vi "test_read-nmea-data2.vi"() -> ()   [LabVIEW 2019] (continued)
104,,19,25,045,,25,08,248,,36,27,309,,2*77\n\t\n15:15:25.65\tF9P\t$GBGSV,2,1,06,07,,,26,11,48,133,32,14,87,101,33,28,,,24,1*7A\n\t\n15:15:25.67\tF9P\t$GBGSV,2,2,06,33,62,220,35,34,,,26,1*41\n\t\n15:15:25.69\tF9P\t$GBGSV,1,1,03,11,48,133,33,14,87,101,29,33,62,220,,3*4F\n\t\n15:15:25.71\tF9P\t$GNGLL,3723.59755,N,12656.93215,E,061527.00,A,A*74\n\t\n15:15:25.73\tF9P\t\t\n15:15:25.75\tF9P\t\t\n15:15:25.77\tF9P\t\t\n15:15:25.79\tF9P\t\t\n15:15:25.81\tF9P\t\t\n15:15:25.83\tF9P\t\t\n15:15:25.85\tF9P\t\t\n15:15:25.87\tF9P\t\t\n15:15:25.89\tF9P\t\t\n15:15:25.91\tF9P\t\t\n15:15:25.93\tF9P\t\t\n15:15:25.95\tF9P\t\t\n15:15:25.97\tF9P\t\t\n15:15:25.99\tF9P\t\t\n15:15:26.01\tF9P\t\t\n15:15:26.03\tF9P\t\t\n15:15:26.05\tF9P\t\t\n15:15:26.07\tF9P\t\t\n15:15:26.09\tF9P\t\t\n15:15:26.11\tF9P\t\t\n15:15:26.13\tF9P\t\t\n15:15:26.15\tF9P\t\t\n15:15:26.17\tF9P\t\t\n15:15:26.19\tF9P\t\t\n15:15:26.21\tF9P\t\t\n15:15:26.23\tF9P\t$GNRMC,061528.00,A,3723.59768,N,12656.93177,E,0.064,,250720,,,A,V*11\n\t\n15:15:26.25\tF9P\t$GNVTG,,T,,M,0.064,N,0.118,K,A*37\n\t\n15:15:26.27\tF9P\t$GNGGA,061528.00,3723.59768,N,12656.93177,E,1,12,0.80,45.8,M,18.5,M,,*79\n\t\n15:15:26.29\tF9P\t$GNGSA,A,3,12,06,19,05,17,09,04,02,,,,,1.41,0.80,1.16,1*0A\n\t\n15:15:26.31\tF9P\t$GNGSA,A,3,85,70,71,84,,,,,,,,,1.41,0.80,1.16,2*08\n\t\n15:15:26.33\tF9P\t$GNGSA,A,3,36,19,11,04,09,12,,,,,,,1.41,0.80,1.16,3*0A\n\t\n15:15:26.35\tF9P\t$GNGSA,A,3,14,11,33,,,,,,,,,,1.41,0.80,1.16,4*0B\n\t\n15:15:26.37\tF9P\t$GPGSV,3,1,09,02,56,320,21,04,17,043,28,05,38,248,29,06,64,051,33,1*68\n\t\n15:15:26.39\tF9P\t$GPGSV,3,2,09,09,44,072,32,12,23,275,40,17,31,154,26,19,51,157,27,1*6D\n\t\n15:15:26.41\tF9P\t$GPGSV,3,3,09,25,12,305,21,1*5C\n\t\n15:15:26.43\tF9P\t$GPGSV,3,1,09,02,56,320,,04,17,043,18,05,38,248,22,06,64,051,30,6*67\n\t\n15:15:26.45\tF9P\t$GPGSV,3,2,09,09,44,072,26,12,23,275,21,17,31,154,,19,51,157,,6*69\n\t\n15:15:26.47\tF9P\t$GPGSV,3,3,09,25,12,305,,6*58\n\t\n15:15:26.49\tF9P\t$GLGSV,2,1,08,69,10,031,21,70,70,037,34,71,54,207,37,72,05,210,,1*7A\n\t\n15:15:26.51\tF9P\t$GLGSV,2,2,08,77,01,324,,84,19,123,10,85,69,072,37,86,38,331,,1*76\n\t\n15:15:26.53\tF9P\t$GLGSV,2,1,08,69,10,031,13,70,70,037,,71,54,207,31,72,05,210,,3*78\n\t\n15:15:26.55\tF9P\t$GLGSV,2,2,08,77,01,324,,84,19,123,11,85,69,072,34,86,38,331,,3*76\n\t\n15:15:26.57\tF9P\t$GAGSV,2,1,08,02,08,296,11,04,67,114,40,09,33,193,28,11,72,002,35,7*73\n\t\n15:15:26.59\tF9P\t$GAGSV,2,2,08,12,39,104,26,19,25,044,26,25,08,248,,36,27,309,18,7*7A\n\t\n15:15:26.61\tF9P\t$GAGSV,2,1,08,02,08,296,,04,67,114,,09,33,193,,11,72,002,33,2*7E\n\t\n15:15:26.63\tF9P\t$GAGSV,2,2,08,12,39,104,,19,25,044,,25,08,248,,36,27,309,,2*76\n\t\n15:15:26.65\tF9P\t$GBGSV,2,1,06,07,,,25,11,48,133,32,14,87,101,35,28,,,24,1*7F\n\t\n15:15:26.67\tF9P\t$GBGSV,2,2,06,33,62,220,36,34,,,26,1*42\n\t\n15:15:26.69\tF9P\t$GBGSV,1,1,03,11,48,133,,14,87,101,23,33,62,220,,3*45\n\t\n15:15:26.71\tF9P\t$GNGLL,3723.59768,N,12656.93177,E,061528.00,A,A*72\n\t\n15:15:26.73\tF9P\t\t\n15:15:26.75\tF9P\t\t\n15:15:26.77\tF9P\t\t\n15:15:26.79\tF9P\t\t\n15:15:26.81\tF9P\t\t\n15:15:26.83\tF9P\t\t\n15:15:26.85\tF9P\t\t\n15:15:26.87\tF9P\t\t\n15:15:26.89\tF9P\t\t\n15:15:26.91\tF9P\t\t\n15:15:26.93\tF9P\t\t\n15:15:26.95\tF9P\t\t\n15:15:26.97\tF9P\t\t\n15:15:26.99\tF9P\t\t\n15:15:27.01\tF9P\t\t\n15:15:27.03\tF9P\t\t\n15:15:27.05\tF9P\t\t\n15:15:27.07\tF9P\t\t\n15:15:27.09\tF9P\t\t\n15:15:27.11\tF9P\t\t\n15:15:27.13\tF9P\t\t\n15:15:27.15\tF9P\t\t\n15:15:27.17\tF9P\t\t\n15:15:27.19\tF9P\t\t\n15:15:27.21\tF9P\t\t\n15:15:27.23\tF9P\t$GNRMC,061529.00,A,3723.59788,N,12656.93143,E,0.112,,250720,,,A,V*19\n\t\n15:15:27.25\tF9P\t$GNVTG,,T,,M,0.112,N,0.208,K,A*35\n\t\n15:15:27.27\tF9P\t$GNGGA,061529.00,3723.59788,N,12656.93143,E,1,12,0.72,45.7,M,18.5,M,,*73\n\t\n15:15:27.29\tF9P\t$GNGSA,A,3,12,06,19,05,17,09,04,02,,,,,1.23,0.72,1.00,1*04\n\t\n15:15:27.31\tF9P\t$GNGSA,A,3,85,70,71,84,,,,,,,,,1.23,0.72,1.00,2*06\n\t\n15:15:27.33\tF9P\t$GNGSA,A,3,36,19,11,04,09,12,,,,,,,1.23,0.72,1.00,3*04\n\t\n15:15:27.35\tF9P\t$GNGSA,A,3,14,11,33,,,,,,,,,,1.23,0.72,1.00,4*05\n\t\n15:15:27.37\tF9P\t$GPGSV,3,1,09,02,56,320,21,04,17,043,28,05,38,248,29,06,64,051,33,1*68\n\t\n15:15:27.39\tF9P\t$GPGSV,3,2,09,09,44,072,36,12,23,275,39,17,31,154,25,19,51,157,27,1*64\n\t\n15:15:27.41\tF9P\t$GPGSV,3,3,09,25,12,305,23,1*5E\n\t\n15:15:27.43\tF9P\t$GPGSV,3,1,09,02,56,320,,04,17,043,18,05,38,248,22,06,64,051,30,6*67\n\t\n15:15:27.45\tF9P\t$GPGSV,3,2,09,09,44,072,27,12,23,275,15,17,31,154,,19,51,157,,6*6F\n\t\n15:15:27.47\tF9P\t$GPGSV,3,3,09,25,12,305,,6*58\n\t\n15:15:27.49\tF9P\t$GLGSV,2,1,08,69,10,031,22,70,70,037,29,71,54,207,30,72,05,210,,1*72\n\t\n15:15:27.51\tF9P\t$GLGSV,2,2,08,77,01,324,,84,19,123,12,85,69,072,38,86,38,331,,1*7B\n\t\n15:15:27.53\tF9P\t$GLGSV,2,1,08,69,10,031,13,70,70,037,,71,54,207,30,72,05,210,,3*79\n\t\n15:15:27.55\tF9P\t$GLGSV,2,2,08,77,01,324,,84,19,123,10,85,69,072,28,86,38,331,,3*7A\n\t\n15:15:27.57\tF9P\t$GAGSV,2,1,08,02,08,296,07,04,67,114,42,09,33,193,28,11,72,002,34,7*77\n\t\n15:15:27.59\tF9P\t$GAGSV,2,2,08,12,39,104,26,19,25,044,25,25,08,248,,36,27,309,11,7*70\n\t\n15:15:27.61\tF9P\t$GAGSV,2,1,08,02,08,296,,04,67,114,30,09,33,193,,11,72,002,32,2*7C\n\t\n15:15:27.63\tF9P\t$GAGSV,2,2,08,12,39,104,,19,25,044,,25,08,248,,36,27,309,,2*76\n\t\n15:15:27.65\tF9P\t$GBGSV,2,1,06,07,,,25,11,48,133,33,14,87,101,31,28,,,20,1*7E\n\t\n15:15:27.67\tF9P\t$GBGSV,2,2,06,33,62,220,38,34,,,27,1*4D\n\t\n15:15:27.69\tF9P\t$GBGSV,1,1,03,11,48,133,,14,87,101,,33,62,220,,3*44\n\t\n15:15:27.71\tF9P\t$GNGLL,3723.59788,N,12656.93143,E,061529.00,A,A*7A\n\t\n15:15:27.73\tF9P\t\t\n15:15:27.75\tF9P\t\t\n15:15:27.77\tF9P\t\t\n15:15:27.79\tF9P\t\t\n15:15:27.81\tF9P\t\t\n15:15:27.83\tF9P\t\t\n15:15:27.85\tF9P\t\t\n15:15:27.87\tF9P\t\t\n15:15:27.89\tF9P\t\t\n15:15:27.91\tF9P\t\t\n15:15:27.93\tF9P\t\t\n15:15:27.95\tF9P\t\t\n15:15:27.97\tF9P\t\t\n15:15:27.99\tF9P\t\t\n15:15:28.01\tF9P\t\t\n15:15:28.03\tF9P\t\t\n15:15:28.05\tF9P\t\t\n15:15:28.07\tF9P\t\t\n15:15:28.09\tF9P\t\t\n15:15:28.11\tF9P\t\t\n15:15:28.13\tF9P\t\t\n15:15:28.15\tF9P\t\t\n15:15:28.17\tF9P\t\t\n15:15:28.19\tF9P\t\t\n15:15:28.21\tF9P\t\t\n15:15:28.23\tF9P\t$GNRMC,061530.00,A,3723.59812,N,12656.93103,E,0.030,,250720,,,A,V*18\n\t\n15:15:28.25\tF9P\t$GNVTG,,T,,M,0.030,N,0.055,K,A*3E\n\t\n15:15:28.27\tF9P\t$GNGGA,061530.00,3723.59812,N,12656.93103,E,1,12,0.71,45.7,M,18.5,M,,*70\n\t\n15:15:28.29\tF9P\t$GNGSA,A,3,12,06,19,05,17,09,04,02,,,,,1.22,0.71,1.00,1*06\n\t\n15:15:28.31\tF9P\t$GNGSA,A,3,85,70,71,84,,,,,,,,,1.22,0.71,1.00,2*04\n\t\n15:15:28.33\tF9P\t$GNGSA,A,3,36,19,11,04,09,12,,,,,,,1.22,0.71,1.00,3*06\n\t\n15:15:28.35\tF9P\t$GNGSA,A,3,14,11,33,,,,,,,,,,1.22,0.71,1.00,4*07\n\t\n15:15:28.37\tF9P\t$GPGSV,3,1,09,02,56,320,20,04,17,043,26,05,38,248,28,06,64,051,33,1*66\n\t\n15:15:28.39\tF9P\t$GPGSV,3,2,09,09,44,072,35,12,23,275,37,17,31,154,24,19,51,157,27,1*68\n\t\n15:15:28.41\tF9P\t$GPGSV,3,3,09,25,12,305,25,1*58\n\t\n15:15:28.43\tF9P\t$GPGSV,3,1,09,02,56,320,,04,17,043,18,05,38,248,22,06,64,051,32,6*65\n\t\n15:15:28.45\tF9P\t$GPGSV,3,2,09,09,44,072,27,12,23,275,16,17,31,154,,19,51,157,,6*6C\n\t\n15:15:28.47\tF9P\t$GPGSV,3,3,09,25,12,305,,6*58\n\t\n15:15:28.49\tF9P\t$GLGSV,2,1,08,69,10,031,22,70,70,037,28,71,54,207,37,72,05,210,,1*74\n\t\n15:15:28.51\tF9P\t$GLGSV,2,2,08,77,01,324,,84,19,123,11,85,69,072,39,86,38,331,,1*79\n\t\n15:15:28.53\tF9P\t$GLGSV,2,1,08,69,10,031,13,70,70,037,,71,54,207,30,72,05,210,,3*79\n\t\n15:15:28.55\tF9P\t$GLGSV,2,2,08,77,01,324,,84,19,123,09,85,69,072,30,86,38,331,,3*7B\n\t\n15:15:28.57\tF9P\t$GAGSV,2,1,08,02,08,296,08,04,67,114,39,09,33,193,33,11,72,002,32,7*78\n\t\n15:15:28.59\tF9P\t$GAGSV,2,2,08,12,39,104,27,19,25,044,22,25,08,248,,36,27,309,13,7*74\n\t\n15:15:28.61\tF9P\t$GAGSV,2,1,08,02,08,296,,04,67,114,34,09,33,193,,11,72,002,32,2*78\n\t\n15:15:28.63\tF9P\t$GAGSV,2,2,08,12,39,104,,19,25,044,,25,08,248,,36,27,309,,2*76\n\t\n15:15:28.65\tF9P\t$GBGSV,2,1,06,07,,,25,11,48,133,32,14,87,101,27,28,,,23,1*7B\n\t\n15:15:28.67\tF9P\t$GBGSV,2,2,06,33,62,220,37,34,,,28,1*4D\n\t\n15:15:28.69\tF9P\t$GBGSV,1,1,03,11,48,133,,14,87,101,,33,62,220,,3*44\n\t\n15:15:28.71\tF9P\t$GNGLL,3723.59812,N,12656.93103,E,061530.00,A,A*7A\n\t\n15:15:28.73\tF9P\t\t\n15:15:28.75\tF9P\t\t\n15:15:28.77\tF9P\t\t\n15:15:28.79\tF9P\t\t\n15:15:28.81\tF9P\t\t\n15:15:28.83\tF9P\t\t\n15:15:28.85\tF9P\t\t\n15:15:28.87\tF9P\t\t\n15:15:28.89\tF9P\t\t\n15:15:28.91\tF9P\t\t\n15:15:28.93\tF9P\t\t\n15:15:28.95\tF9P\t\t\n15:15:28.97\tF9P\t\t\n15:15:28.99\tF9P\t\t\n15:15:29.01\tF9P\t\t\n15:15:29.03\tF9P\t\t\n15:15:29.05\tF9P\t\t\n15:15:29.07\tF9P\t\t\n15:15:29.09\tF9P\t\t\n15:15:29.11\tF9P\t\t\n15:15:29.13\tF9P\t\t\n15:15:29.15\tF9P\t\t\n15:15:29.17\tF9P\t\t\n15:15:29.19\tF9P\t\t\n15:15:29.21\tF9P\t\t\n15:15:29.23\tF9P\t$GNRMC,061531.00,A,3723.59835,N,12656.93068,E,0.052,,250720,,,A,V*14\n\t\n15:15:29.25\tF9P\t$GNVTG,,T,,M,0.052,N,0.096,K,A*35\n\t\n15:15:29.27\tF9P\t$GNGGA,061531.00,3723.59835,N,12656.93068,E,1,12,0.71,45.6,M,18.5,M,,*79\n\t\n15:15:29.29\tF9P\t$GNGSA,A,3,12,06,19,05,17,09,04,02,,,,,1.22,0.71,1.00,1*06\n\t\n15:15:29.31\tF9P\t$GNGSA,A,3,85,70,71,84,,,,,,,,,1.22,0.71,1.00,2*04\n\t\n15:15:29.33\tF9P\t$GNGSA,A,3,36,19,11,04,09,12,,,,,,,1.22,0.71,1.00,3*06\n\t\n15:15:29.35\tF9P\t$GNGSA,A,3,14,11,33,,,,,,,,,,1.22,0.71,1.00,4*07\n\t\n15:15:29.37\tF9P\t$GPGSV,3,1,09,02,56,320,19,04,17,043,27,05,38,248,20,06,64,051,37,1*61\n\t\n15:15:29.39\tF9P\t$GPGSV,3,2,09,09,44,072,26,12,23,275,37,17,31,154,22,19,51,157,27,1*6C\n\t\n15:15:29.41\tF9P\t$GPGSV,3,3,09,25,12,305,25,1*58\n\t\n15:15:29.43\tF9P\t$GPGSV,3,1,09,02,56,320,,04,17,043,19,05,38,248,23,06,64,051,34,6*63\n\t\n15:15:29.45\tF9P\t$GPGSV,3,2,09,09,44,072,27,12,23,275,21,17,31,154,,19,51,157,,6*68\n\t\n15:15:29.47\tF9P\t$GPGSV,3,3,09,25,12,305,,6*58\n\t\n15:15:29.49\tF9P\t$GLGSV,2,1,08,69,10,031,25,70,70,037,32,71,54,207,37,72,05,210,,1*78\n\t\n15:15:29.51\tF9P\t$GLGSV,2,2,08,77,01,324,,84,19,123,11,85,69,072,40,86,38,331,,1*77\n\t\n15:15:29.53\tF9P\t$GLGSV,2,1,08,69,10,031,10,70,70,037,,71,54,207,29,72,05,210,,3*72\n\t\n15:15:29.55\tF9P\t$GLGSV,2,2,08,77,01,324,,84,19,123,12,85,69,072,32,86,38,331,,3*73\n\t\n15:15:29.57\tF9P\t$GAGSV,2,1,08,02,08,296,08,04,67,114,39,09,33,193,30,11,72,002,32,7*7B\n\t\n15:15:29.59\tF9P\t$GAGSV,2,2,08,12,39,104,27,19,25,044,22,25,08,248,,36,27,309,14,7*73\n\t\n15:15:29.61\tF9P\t$GAGSV,2,1,08,02,08,296,,04,67,114,29,09,33,193,,11,72,002,32,2*74\n\t\n15:15:29.63\tF9P\t$GAGSV,2,2,08,12,39,104,,19,25,044,,25,08,248,,36,27,309,,2*76\n\t\n15:15:29.65\tF9P\t$GBGSV,2,1,06,07,,,25,11,48,133,31,14,87,101,30,28,,,23,1*7E\n\t\n15:15:29.67\tF9P\t$GBGSV,2,2,06,33,62,220,37,34,,,28,1*4D\n\t\n15:15:29.69\tF9P\t$GBGSV,1,1,03,11,48,133,,14,87,101,,33,62,220,,3*44\n\t\n15:15:29.71\tF9P\t$GNGLL,3723.59835,N,12656.93068,E,061531.00,A,A*72\n\t\n15:15:29.73\tF9P\t\t\n15:15:29.75\tF9P\t\t\n15:15:29.77\tF9P\t\t\n15:15:29.79\tF9P\t\t\n15:15:29.81\tF9P\t\t\n15:15:29.83\tF9P\t\t\n15:15:29.85\tF9P\t\t\n15:15:29.87\tF9P\t\t\n15:15:29.89\tF9P\t\t\n15:15:29.91\tF9P\t\t\n15:15:29.93\tF9P\t\t\n15:15:29.95\tF9P\t\t\n15:15:29.97\tF9P\t\t\n15:15:29.99\tF9P\t\t\n15:15:30.01\tF9P\t\t\n15:15:30.03\tF9P\t\t\n15:15:30.05\tF9P\t\t\n15:15:30.07\tF9P\t\t\n15:15:30.09\tF9P\t\t\n15:15:30.11\tF9P\t\t\n15:15:30.13\tF9P\t\t\n15:15:30.15\tF9P\t\t\n15:15:30.17\tF9P\t\t\n15:15:30.19\tF9P\t\t\n15:15:30.21\tF9P\t\t\n15:15:30.23\tF9P\t$GNRMC,061532.00,A,3723.59857,N,12656.93043,E,0.021,,250720,,,A,V*1E\n\t\n15:15:30.25\tF9P\t$GNVTG,,T,,M,0.021,N,0.040,K,A*3A\n\t\n15:15:30.27\tF9P\t$GNGGA,061532.00,3723.59857,N,12656.93043,E,1,12,0.71,45.7,M,18.5,M,,*76\n\t\n15:15:30.29\tF9P\t$GNGSA,A,3,12,06,19,05,17,09,04,02,,,,,1.22,0.71,1.00,1*06\n\t\n15:15:30.31\tF9P\t$GNGSA,A,3,85,70,71,84,,,,,,,,,1.22,0.71,1.00,2*04\n\t\n15:15:30.33\tF9P\t$GNGSA,A,3,36,19,11,04,09,12,,,,,,,1.22,0.71,1.00,3*06\n\t\n15:15:30.35\tF9P\t$GNGSA,A,3,14,11,33,,,,,,,,,,1.22,0.71,1.00,4*07\n\t\n15:15:30.37\tF9P\t$GPGSV,3,1,09,02,56,320,21,04,17,043,28,05,38,248,30,06,64,051,36,1*65\n\t\n15:15:30.39\tF9P\t$GPGSV,3,2,09,09,44,072,25,12,23,275,36,17,31,154,19,19,51,157,29,1*68\n\t\n15:15:30.41\tF9P\t$GPGSV,3,3,09,25,12,305,26,1*5B\n\t\n15:15:30.43\tF9P\t$GPGSV,3,1,09,02,56,320,,04,17,043,18,05,38,248,23,06,64,051,33,6*65\n\t\n15:15:30.45\tF9P\t$GPGSV,3,2,09,09,44,072,27,12,23,275,24,17,31,154,,19,51,157,,6*6D\n\t\n15:15:30.47\tF9P\t$GPGSV,3,3,09,25,12,305,,6*58\n\t\n15:15:30.49\tF9P\t$GLGSV,2,1,08,69,10,031,28,70,70,037,33,71,54,207,33,72,05,210,,1*70\n\t\n15:15:30.51\tF9P\t$GLGSV,2,2,08,77,01,324,,84,19,123,11,85,69,072,40,86,38,331,,1*77\n\t\n15:15:30.53\tF9P\t$GLGSV,2,1,08,69,10,031,08,70,70,037,,71,54,207,29,72,05,210,,3*7B\n\t\n15:15:30.55\tF9P\t$GLGSV,2,2,08,77,01,324,,84,19,123,16,85,69,072,33,86,38,331,,3*76\n\t\n15:15:30.57\tF9P\t$GAGSV,2,1,08,02,08,296,11,04,67,114,39,09,33,193,32,11,72,002,31,7*72\n\t\n15:15:30.59\tF9P\t$GAGSV,2,2,08,12,39,104,27,19,25,044,21,25,08,248,,36,27,309,13,7*77\n\t\n15:15:30.61\tF9P\t$GAGSV,2,1,08,02,08,296,,04,67,114,27,09,33,193,27,11,72,002,33,2*7E\n\t\n15:15:30.63\tF9P\t$GAGSV,2,2,08,12,39,104,,19,25,044,,25,08,248,,36,27,309,,2*76\n\t\n15:15:30.65\tF9P\t$GBGSV,2,1,06,07,,,23,11,48,133,30,14,87,101,31,28,,,25,1*7E\n\t\n15:15:30.67\tF9P\t$GBGSV,2,2,06,33,62,220,38,34,,,28,1*42\n\t\n15:15:30.69\tF9P\t$GBGSV,1,1,03,11,48,133,,14,87,101,,33,62,220,,3*44\n\t\n15:15:30.71\tF9P\t$GNGLL,3723.59857,N,12656.93043,E,061532.00,A,A*7C\n\t\n15:15:30.73\tF9P\t\t\n15:15:30.75\tF9P\t\t\n15:15:30.77\tF9P\t\t\n15:15:30.79\tF9P\t\t\n15:15:30.81\tF9P\t\t\n15:15:30.83\tF9P\t\t\n15:15:30.85\tF9P\t\t\n15:15:30.87\tF9P\t\t\n15:15:30.89\tF9P\t\t\n15:15:30.91\tF9P\t\t\n15:15:30.93\tF9P\t\t\n15:15:30.95\tF9P\t\t\n15:15:30.97\tF9P\t\t\n15:15:30.99\tF9P\t\t\n15:15:31.01\tF9P\t\t\n15:15:31.03\tF9P\t\t\n15:15:31.05\tF9P\t\t\n15:15:31.07\tF9P\t\t\n15:15:31.09\tF9P\t\t\n15:15:31.11\tF9P\t\t\n15:15:31.13\tF9P\t\t\n15:15:31.15\tF9P\t\t\n15:15:31.17\tF9P\t\t\n15:15:31.19\tF9P\t\t\n15:15:31.21\tF9P\t\t\n15:15:31.23\tF9P\t$GNRMC,061533.00,A,3723.59881,N,12656.93016,E,0.059,,250720,,,A,V*1B\n\t\n15:15:31.25\tF9P\t$GNVTG,,T,,M,0.059,N,0.110,K,A*31\n\t\n15:15:31.27\tF9P\t$GNGGA,061533.00,3723.59881,N,12656.93016,E,1,12,0.71,45.8,M,18.5,M,,*73\n\t\n15:15:31.29\tF9P\t$GNGSA,A,3,12,06,19,05,17,09,04,02,,,,,1.22,0.71,1.00,1*06\n\t\n15:15:31.31\tF9P\t$GNGSA,A,3,85,70,71,84,,,,,,,,,1.22,0.71,1.00,2*04\n\t\n15:15:31.33\tF9P\t$GNGSA,A,3,36,19,11,04,09,12,,,,,,,1.22,0.71,1.00,3*06\n\t\n15:15:31.35\tF9P\t$GNGSA,A,3,14,11,33,,,,,,,,,,1.22,0.71,1.00,4*07\n\t\n15:15:31.37\tF9P\t$GPGSV,3,1,09,02,56,320,22,04,17,043,27,05,38,248,30,06,64,051,35,1*6A\n\t\n15:15:31.39\tF9P\t$GPGSV,3,2,09,09,44,072,26,12,23,275,38,17,31,154,20,19,51,157,28,1*6E\n\t\n15:15:31.41\tF9P\t$GPGSV,3,3,09,25,12,305,26,1*5B\n\t\n15:15:31.43\tF9P\t$GPGSV,3,1,09,02,56,320,,04,17,043,18,05,38,248,23,06,64,051,33,6*65\n\t\n15:15:31.45\tF9P\t$GPGSV,3,2,09,09,44,072,28,12,23,275,24,17,31,154,,19,51,157,,6*62\n\t\n15:15:31.47\tF9P\t$GPGSV,3,3,09,25,12,305,,6*58\n\t\n15:15:31.49\tF9P\t$GLGSV,2,1,08,69,10,031,26,70,70,037,31,71,54,207,32,72,05,210,,1*7D\n\t\n15:15:31.51\tF9P\t$GLGSV,2,2,08,77,01,324,,84,19,123,11,85,69,072,38,86,38,331,,1*78\n\t\n15:15:31.53\tF9P\t$GLGSV,2,1,08,69,10,031,07,70,70,037,,71,54,207,26,72,05,210,,3*7B\n\t\n15:15:31.55\tF9P\t$GLGSV,2,2,08,77,01,324,,84,19,123,11,85,69,072,33,86,38,331,,3*71\n\t\n15:15:31.57\tF9P\t$GAGSV,2,1,08,02,08,296,10,04,67,114,39,09,33,193,34,11,72,002,30,7*74\n\t\n15:15:31.59\tF9P\t$GAGSV,2,2,08,12,39,104,26,19,25,044,24,25,08,248,,36,27,309,16,7*76\n\t\n15:15:31.61\tF9P\t$GAGSV,2,1,08,02,08,296,,04,67,114,,09,33,193,28,11,72,002,33,2*74\n\t\n15:15:31.63\tF9P\t$GAGSV,2,2,08,12,39,104,,19,25,044,,25,08,248,,36,27,309,,2*76\n\t\n15:15:31.65\tF9P\t$GBGSV,2,1,06,07,,,21,11,48,133,28,14,87,101,29,28,,,25,1*7C\n\t\n15:15:31.67\tF9P\t$GBGSV,2,2,06,33,62,220,38,34,,,27,1*4D\n\t\n15:15:31.69\tF9P\t$GBGSV,1,1,03,11,48,133,,14,87,101,,33,62,220,,3*44\n\t\n15:15:31.71\tF9P\t$GNGLL,3723.59881,N,12656.93016,E,061533.00,A,A*76\n\t\n15:15:31.73\tF9P\t\t\n15:15:31.75\tF9P\t\t\n15:15:31.77\tF9P\t\t\n15:15:31.79\tF9P\t\t\n15:15:31.81\tF9P\t\t\n15:15:31.83\tF9P\t\t\n15:15:31.85\tF9P\t\t\n15:15:31.87\tF9P\t\t\n15:15:31.89\tF9P\t\t\n15:15:31.91\tF9P\t\t\n15:15:31.93\tF9P\t\t\n15:15:31.95\tF9P\t\t\n15:15:31.97\tF9P\t\t\n15:15:31.99\tF9P\t\t\n15:15:32.01\tF9P\t\t\n15:15:32.03\tF9P\t\t\n15:15:32.05\tF9P\t\t\n15:15:32.07\tF9P\t\t\n15:15:32.09\tF9P\t\t\n15:15:32.11\tF9P\t\t\n15:15:32.13\tF9P\t\t\n15:15:32.15\tF9P\t\t\n15:15:32.17\tF9P\t\t\n15:15:32.19\tF9P\t\t\n15:15:32.21\tF9P\t\t\n15:15:32.23\tF9P\t$GNRMC,061534.00,A,3723.59903,N,12656.92993,E,0.051,,250720,,,A,V*1A\n\t\n15:15:32.25\tF9P\t$GNVTG,,T,,M,0.051,N,0.095,K,A*35\n\t\n15:15:32.27\tF9P\t$GNGGA,061534.00,3723.59903,N,12656.92993,E,1,12,0.71,45.9,M,18.5,M,,*7B\n\t\n15:15:32.29\tF9P\t$GNGSA,A,3,12,06,19,05,17,09,04,02,,,,,1.22,0.71,1.00,1*06\n\t\n15:15:32.31\tF9P\t$GNGSA,A,3,85,70,71,84,,,,,,,,,1.22,0.71,1.00,2*04\n\t\n15:15:32.33\tF9P\t$GNGSA,A,3,36,19,11,04,09,12,,,,,,,1.22,0.71,1.00,3*06\n\t\n15:15:32.35\tF9P\t$GNGSA,A,3,14,11,33,,,,,,,,,,1.22,0.71,1.00,4*07\n\t\n15:15:32.37\tF9P\t$GPGSV,3,1,09,02,56,320,23,04,17,043,27,05,38,248,29,06,64,051,37,1*61\n\t\n15:15:32.39\tF9P\t$GPGSV,3,2,09,09,44,072,26,12,23,275,38,17,31,154,21,19,51,157,27,1*60\n\t\n15:15:32.41\tF9P\t$GPGSV,3,3,09,25,12,305,26,1*5B\n\t\n15:15:32.43\tF9P\t$GPGSV,3,1,09,02,56,320,,04,17,043,17,05,38,248,23,06,64,051,34,6*6D\n\t\n15:15:32.45\tF9P\t$GPGSV,3,2,09,09,44,072,27,12,23,275,22,17,31,154,20,19,51,157,,6*69\n\t\n15:15:32.47\tF9P\t$GPGSV,3,3,09,25,12,305,,6*58\n\t\n15:15:32.49\tF9P\t$GLGSV,2,1,08,69,10,031,26,70,70,037,29,71,54,207,32,72,05,210,,1*74\n\t\n15:15:32.51\tF9P\t$GLGSV,2,2,08,77,01,324,,84,19,123,10,85,69,072,36,86,38,331,,1*77\n\t\n15:15:32.53\tF9P\t$GLGSV,2,1,08,69,10,031,,70,70,037,,71,54,207,26,72,05,210,,3*7C\n\t\n15:15:32.55\tF9P\t$GLGSV,2,2,08,77,01,324,,84,19,123,10,85,69,072,33,86,38,331,,3*70\n\t\n15:15:32.57\tF9P\t$GAGSV,2,1,08,02,08,296,09,04,67,114,39,09,33,193,34,11,72,002,31,7*7D\n\t\n15:15:32.59\tF9P\t$GAGSV,2,2,08,12,39,104,26,19,25,044,25,25,08,248,,36,27,309,17,7*76\n\t\n15:15:32.61\tF9P\t$GAGSV,2,1,08,02,08,296,,04,67,114,,09,33,193,28,11,72,002,33,2*74\n\t\n15:15:32.63\tF9P\t$GAGSV,2,2,08,12,39,104,,19,25,044,,25,08,248,,36,27,309,,2*76\n\t\n15:15:32.65\tF9P\t$GBGSV,2,1,06,07,,,21,11,48,133,28,14,87,101,30,28,,,25,1*74\n\t\n15:15:32.67\tF9P\t$GBGSV,2,2,06,33,62,220,38,34,,,27,1*4D\n\t\n15:15:32.69\tF9P\t$GBGSV,1,1,03,11,48,133,,14,87,101,,33,62,220,,3*44\n\t\n15:15:32.71\tF9P\t$GNGLL,3723.59903,N,12656.92993,E,061534.00,A,A*7F\n\t\n15:15:32.73\tF9P\t\t\n15:15:32.75\tF9P\t\t\n15:15:32.77\tF9P\t\t\n15:15:32.79\tF9P\t\t\n15:15:32.81\tF9P\t\t\n15:15:32.83\tF9P\t\t\n15:15:32.85\tF9P\t\t\n15:15:32.87\tF9P\t\t\n15:15:32.89\tF9P\t\t\n15:15:32.91\tF9P\t\t\n15:15:32.93\tF9P\t\t\n15:15:32.95\tF9P\t\t\n15:15:32.97\tF9P\t\t\n15:15:32.99\tF9P\t\t\n15:15:33.01\tF9P\t\t\n15:15:33.03\tF9P\t\t\n15:15:33.05\tF9P\t\t\n15:15:33.07\tF9P\t\t\n15:15:33.09\tF9P\t\t\n15:15:33.11\tF9P\t\t\n15:15:33.13\tF9P\t\t\n15:15:33.15\tF9P\t\t\n15:15:33.17\tF9P\t\t\n15:15:33.19\tF9P\t\t\n15:15:33.21\tF9P\t\t\n15:15:33.23\tF9P\t$GNRMC,061535.00,A,3723.59921,N,12656.92973,E,0.029,,250720,,,A,V*1A\n\t\n15:15:33.25\tF9P\t$GNVTG,,T,,M,0.029,N,0.053,K,A*30\n\t\n15:15:33.27\tF9P\t$GNGGA,061535.00,3723.59921,N,12656.92973,E,1,12,0.71,46.0,M,18.5,M,,*7E\n\t\n15:15:33.29\tF9P\t$GNGSA,A,3,12,06,19,05,17,09,04,02,,,,,1.22,0.71,1.00,1*06\n\t\n15:15:33.31\tF9P\t$GNGSA,A,3,85,70,71,84,,,,,,,,,1.22,0.71,1.00,2*04\n\t\n15:15:33.33\tF9P\t$GNGSA,A,3,36,19,11,04,09,12,,,,,,,1.22,0.71,1.00,3*06\n\t\n15:15:33.35\tF9P\t$GNGSA,A,3,14,11,33,,,,,,,,,,1.22,0.71,1.00,4*07\n\t\n15:15:33.37\tF9P\t$GPGSV,3,1,09,02,56,320,21,04,17,043,26,05,38,248,29,06,64,051,37,1*62\n\t\n15:15:33.39\tF9P\t$GPGSV,3,2,09,09,44,072,31,12,23,275,38,17,31,154,25,19,51,157,27,1*62\n\t\n15:15:33.41\tF9P\t$GPGSV,3,3,09,25,12,305,26,1*5B\n\t\n15:15:33.43\tF9P\t$GPGSV,3,1,09,02,56,320,,04,17,043,17,05,38,248,23,06,64,051,34,6*6D\n\t\n15:15:33.45\tF9P\t$GPGSV,3,2,09,09,44,072,28,12,23,275,22,17,31,154,18,19,51,157,,6*6D\n\t\n15:15:33.47\tF9P\t$GPGSV,3,3,09,25,12,305,,6*58\n\t\n15:15:33.49\tF9P\t$GLGSV,2,1,08,69,10,031,26,70,70,037,29,71,54,207,27,72,05,210,,1*70\n\t\n15:15:33.51\tF9P\t$GLGSV,2,2,08,77,01,324,,84,19,123,09,85,69,072,37,86,38,331,,1*7E\n\t\n15:15:33.53\tF9P\t$GLGSV,2,1,08,69,10,031,,70,70,037,,71,54,207,26,72,05,210,,3*7C\n\t\n15:15:33.55\tF9P\t$GLGSV,2,2,08,77,01,324,,84,19,123,14,85,69,072,33,86,38,331,,3*74\n\t\n15:15:33.57\tF9P\t$GAGSV,2,1,08,02,08,296,12,04,67,114,38,09,33,193,34,11,72,002,31,7*76\n\t\n15:15:33.59\tF9P\t$GAGSV,2,2,08,12,39,104,25,19,25,044,25,25,08,248,,36,27,309,19,7*7B\n\t\n15:15:33.61\tF9P\t$GAGSV,2,1,08,02,08,296,,04,67,114,,09,33,193,27,11,72,002,33,2*7B\n\t\n15:15:33.63\tF9P\t$GAGSV,2,2,08,12,39,104,,19,25,044,,25,08,248,,36,27,309,,2*76\n\t\n15:15:33.65\tF9P\t$GBGSV,2,1,06,07,,,21,11,48,133,27,14,87,101,29,28,,,24,1*72\n\t\n15:15:33.67\tF9P\t$GBGSV,2,2,06,33,62,220,37,34,,,28,1*4D\n\t\n15:15:33.69\tF9P\t$GBGSV,1,1,03,11,48,133,,14,87,101,,33,62,220,,3*44\n\t\n15:15:33.71\tF9P\t$GNGLL,3723.59921,N,12656.92973,E,061535.00,A,A*70\n\t\n15:15:33.73\tF9P\t\t\n15:15:33.75\tF9P\t\t\n15:15:33.77\tF9P\t\t\n15:15:33.79\tF9P\t\t\n15:15:33.81\tF9P\t\t\n15:15:33.83\tF9P\t\t\n15:15:33.85\tF9P\t\t\n15:15:33.87\tF9P\t\t\n15:15:33.89\tF9P\t\t\n15:15:33.91\tF9P\t\t\n15:15:33.93\tF9P\t\t\n15:15:33.95\tF9P\t\t\n15:15:33.97\tF9P\t\t\n15:15:33.99\tF9P\t\t\n15:15:34.01\tF9P\t\t\n15:15:34.03\tF9P\t\t\n15:15:34.05\tF9P\t\t\n15:15:34.07\tF9P\t\t\n15:15:34.09\tF9P\t\t\n15:15:34.11\tF9P\t\t\n15:15:34.13\tF9P\t\t\n15:15:34.15\tF9P\t\t\n15:15:34.17\tF9P\t\t\n15:15:34.19\tF9P\t\t\n15:15:34.21\tF9P\t\t\n15:15:34.23\tF9P\t$GNRMC,061536.00,A,3723.59940,N,12656.92954,E,0.030,,250720,,,A,V*13\n\t\n15:15:34.25\tF9P\t$GNVTG,,T,,M,0.030,N,0.056,K,A*3D\n\t\n15:15:34.27\tF9P\t$GNGGA,061536.00,3723.59940,N,12656.92954,E,1,12,0.71,46.1,M,18.5,M,,*7E\n\t\n15:15:34.29\tF9P\t$GNGSA,A,3,12,06,19,05,17,09,04,02,,,,,1.22,0.71,1.00,1*06\n\t\n15:15:34.31\tF9P\t$GNGSA,A,3,85,70,71,84,,,,,,,,,1.22,0.71,1.00,2*04\n\t\n15:15:34.33\tF9P\t$GNGSA,A,3,36,19,11,04,09,12,,,,,,,1.22,0.71,1.00,3*06\n\t\n15:15:34.35\tF9P\t$GNGSA,A,3,14,11,33,,,,,,,,,,1.22,0.71,1.00,4*07\n\t\n15:15:34.37\tF9P\t$GPGSV,3,1,09,02,56,320,18,04,17,043,26,05,38,248,30,06,64,051,37,1*60\n\t\n15:15:34.39\tF9P\t$GPGSV,3,2,09,09,44,072,24,12,23,275,38,17,31,154,26,19,51,157,26,1*64\n\t\n15:15:34.41\tF9P\t$GPGSV,3,3,09,25,12,305,26,1*5B\n\t\n15:15:34.43\tF9P\t$GPGSV,3,1,09,02,56,320,,04,17,043,16,05,38,248,23,06,64,051,34,6*6C\n\t\n15:15:34.45\tF9P\t$GPGSV,3,2,09,09,44,072,28,12,23,275,21,17,31,154,15,19,51,157,,6*63\n\t\n15:15:34.47\tF9P\t$GPGSV,3,3,09,25,12,305,,6*58\n\t\n15:15:34.49\tF9P\t$GLGSV,2,1,08,69,10,031,26,70,70,037,29,71,54,207,28,72,05,210,,1*7F\n\t\n15:15:34.51\tF9P\t$GLGSV,2,2,08,77,01,324,,84,19,123,09,85,69,072,37,86,38,331,,1*7E\n\t\n15:15:34.53\tF9P\t$GLGSV,2,1,08,69,10,031,,70,70,037,,71,54,207,26,72,05,210,,3*7C\n\t\n15:15:34.55\tF9P\t$GLGSV,2,2,08,77,01,324,,84,19,123,10,85,69,072,32,86,38,331,,3*71\n\t\n15:15:34.57\tF9P\t$GAGSV,2,1,08,02,08,296,12,04,67,114,38,09,33,193,34,11,72,002,32,7*75\n\t\n15:15:34.59\tF9P\t$GAGSV,2,2,08,12,39,104,25,19,25,044,25,25,08,248,,36,27,309,19,7*7B\n\t\n15:15:34.61\tF9P\t$GAGSV,2,1,08,02,08,296,,04,67,114,,09,33,193,27,11,72,002,33,2*7B\n\t\n15:15:34.63\tF9P\t$GAGSV,2,2,08,12,39,104,,19,25,044,,25,08,248,,36,27,309,,2*76\n\t\n15:15:34.65\tF9P\t$GBGSV,2,1,06,07,,,21,11,48,133,27,14,87,101,30,28,,,23,1*7D\n\t\n15:15:34.67\tF9P\t$GBGSV,2,2,06,33,62,220,36,34,,,28,1*4C\n\t\n15:15:34.69\tF9P\t$GBGSV,1,1,03,11,48,133,,14,87,101,,33,62,220,,3*44\n\t\n15:15:34.71\tF9P\t$GNGLL,3723.59940,N,12656.92954,E,061536.00,A,A*71\n\t\n15:15:34.73\tF9P\t\t\n15:15:34.75\tF9P\t\t\n15:15:34.77\tF9P\t\t\n15:15:34.79\tF9P\t\t\n15:15:34.81\tF9P\t\t\n15:15:34.83\tF9P\t\t\n15:15:34.85\tF9P\t\t\n15:15:34.87\tF9P\t\t\n15:15:34.89\tF9P\t\t\n15:15:34.91\tF9P\t\t\n15:15:34.93\tF9P\t\t\n15:15:34.95\tF9P\t\t\n15:15:34.97\tF9P\t\t\n15:15:34.99\tF9P\t\t\n15:15:35.01\tF9P\t\t\n15:15:35.03\tF9P\t\t\n15:15:35.05\tF9P\t\t\n15:15:35.07\tF9P\t\t\n15:15:35.09\tF9P\t\t\n15:15:35.11\tF9P\t\t\n15:15:35.13\tF9P\t\t\n15:15:35.15\tF9P\t\t\n15:15:35.17\tF9P\t\t\n15:15:35.19\tF9P\t\t\n15:15:35.21\tF9P\t\t\n15:15:35.23\tF9P\t$GNRMC,061537.00,A,3723.59965,N,12656.92930,E,0.006,,250720,,,A,V*12\n\t\n15:15:35.25\tF9P\t$GNVTG,,T,,M,0.006,N,0.012,K,A*38\n\t\n15:15:35.27\tF9P\t$GNGGA,061537.00,3723.59965,N,12656.92930,E,1,12,0.72,46.4,M,18.5,M,,*7C\n\t\n15:15:35.29\tF9P\t$GNGSA,A,3,12,06,19,05,17,09,04,02,,,,,1.21,0.72,0.98,1*06\n\t\n15:15:35.31\tF9P\t$GNGSA,A,3,85,70,71,84,,,,,,,,,1.21,0.72,0.98,2*04\n\t\n15:15:35.33\tF9P\t$GNGSA,A,3,36,19,11,04,09,12,,,,,,,1.21,0.72,0.98,3*06\n\t\n15:15:35.35\tF9P\t$GNGSA,A,3,14,11,33,,,,,,,,,,1.21,0.72,0.98,4*07\n\t\n15:15:35.37\tF9P\t$GPGSV,3,1,09,02,56,320,17,04,17,043,25,05,38,248,29,06,64,051,37,1*64\n\t\n15:15:35.39\tF9P\t$GPGSV,3,2,09,09,44,072,23,12,23,275,38,17,31,154,27,19,51,157,24,1*60\n\t\n15:15:35.41\tF9P\t$GPGSV,3,3,09,25,12,305,24,1*59\n\t\n15:15:35.43\tF9P\t$GPGSV,3,1,09,02,56,320,,04,17,043,17,05,38,248,23,06,64,051,34,6*6D\n\t\n15:15:35.45\tF9P\t$GPGSV,3,2,09,09,44,072,28,12,23,275,20,17,31,154,14,19,51,157,,6*63\n\t\n15:15:35.47\tF9P\t$GPGSV,3,3,09,25,12,305,,6*58\n\t\n15:15:35.50\tF9P\t$GLGSV,2,1,08,69,10,031,25,70,70,037,29,71,54,207,29,72,05,210,,1*7D\n\t\n15:15:35.52\tF9P\t$GLGSV,2,2,08,77,01,324,,84,19,123,13,85,69,072,38,86,38,331,,1*7A\n\t\n15:15:35.54\tF9P\t$GLGSV,2,1,08,69,10,031,,70,70,037,,71,54,207,25,72,05,210,,3*7F\n\t\n15:15:35.56\tF9P\t$GLGSV,2,2,08,77,01,324,,84,19,123,10,85,69,072,33,86,38,331,,3*70\n\t\n15:15:35.58\tF9P\t$GAGSV,2,1,08,02,08,296,15,04,67,114,38,09,33,193,34,11,72,002,31,7*71\n\t\n15:15:35.60\tF9P\t$GAGSV,2,2,08,12,39,104,26,19,25,044,25,25,08,248,,36,27,309,18,7*79\n\t\n15:15:35.62\tF9P\t$GAGSV,2,1,08,02,08,296,,04,67,114,,09,33,193,27,11,72,002,33,2*7B\n\t\n15:15:35.64\tF9P\t$GAGSV,2,2,08,12,39,104,,19,25,044,,25,08,248,,36,27,309,,2*76\n\t\n15:15:35.66\tF9P\t$GBGSV,2,1,06,07,,,21,11,48,133,28,14,87,101,30,28,,,23,1*72\n\t\n15:15:35.68\tF9P\t$GBGSV,2,2,06,33,62,220,37,34,,,28,1*4D\n\t\n15:15:35.70\tF9P\t$GBGSV,1,1,03,11,48,133,,14,87,101,,33,62,220,,3*44\n\t\n15:15:35.72\tF9P\t$GNGLL,3723.59965,N,12656.92930,E,061537.00,A,A*75\n\t\n15:15:35.74\tF9P\t\t\n15:15:35.76\tF9P\t\t\n15:15:35.78\tF9P\t\t\n15:15:35.80\tF9P\t\t\n15:15:35.82\tF9P\t\t\n15:15:35.84\tF9P\t\t\n15:15:35.86\tF9P\t\t\n15:15:35.88\tF9P\t\t\n15:15:35.90\tF9P\t\t\n15:15:35.92\tF9P\t\t\n15:15:35.94\tF9P\t\t\n15:15:35.96\tF9P\t\t\n15:15:35.98\tF9P\t\t\n15:15:36.00\tF9P\t\t\n15:15:36.02\tF9P\t\t\n15:15:36.04\tF9P\t\t\n15:15:36.06\tF9P\t\t\n15:15:36.08\tF9P\t\t\n15:15:36.10\tF9P\t\t\n15:15:36.12\tF9P\t\t\n15:15:36.14\tF9P\t\t\n15:15:36.16\tF9P\t\t\n15:15:36.18\tF9P\t\t\n15:15:36.20\tF9P\t\t\n15:15:36.22\tF9P\t\t\n15:15:36.24\tF9P\t$GNRMC,061538.00,A,3723.59988,N,12656.92906,E,0.049,,250720,,,A,V*10\n\t\n15:15:36.26\tF9P\t$GNVTG,,T,,M,0.049,N,0.091,K,A*38\n\t\n15:15:36.28\tF9P\t$GNGGA,061538.00,3723.59988,N,12656.92906,E,1,12,0.72,46.8,M,18.5,M,,*79\n\t\n15:15:36.30\tF9P\t$GNGSA,A,3,12,06,19,05,17,09,04,02,,,,,1.21,0.72,0.98,1*06\n\t\n15:15:36.32\tF9P\t$GNGSA,A,3,85,70,71,84,,,,,,,,,1.21,0.72,0.98,2*04\n\t\n15:15:36.34\tF9P\t$GNGSA,A,3,36,19,11,04,09,12,,,,,,,1.21,0.72,0.98,3*06\n\t\n15:15:36.36\tF9P\t$GNGSA,A,3,14,11,33,,,,,,,,,,1.21,0.72,0.98,4*07\n\t\n15:15:36.38\tF9P\t$GPGSV,3,1,09,02,56,320,18,04,17,043,26,05,38,248,29,06,64,051,37,1*68\n\t\n15:15:36.40\tF9P\t$GPGSV,3,2,09,09,44,072,21,12,23,275,38,17,31,154,27,19,51,157,23,1*65\n\t\n"
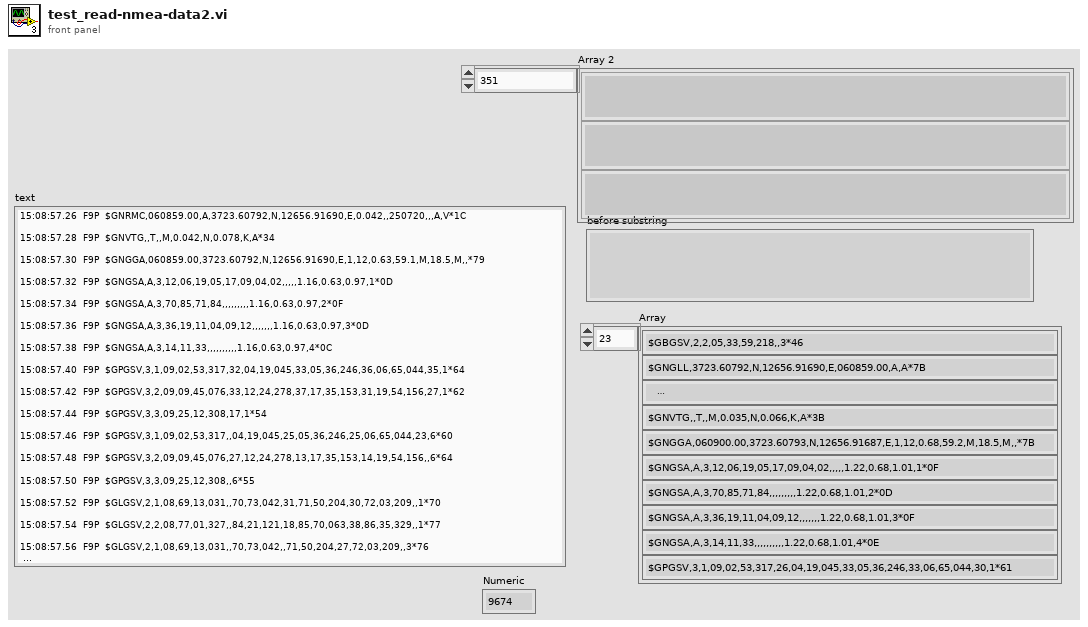
[diagram p1: front panel]
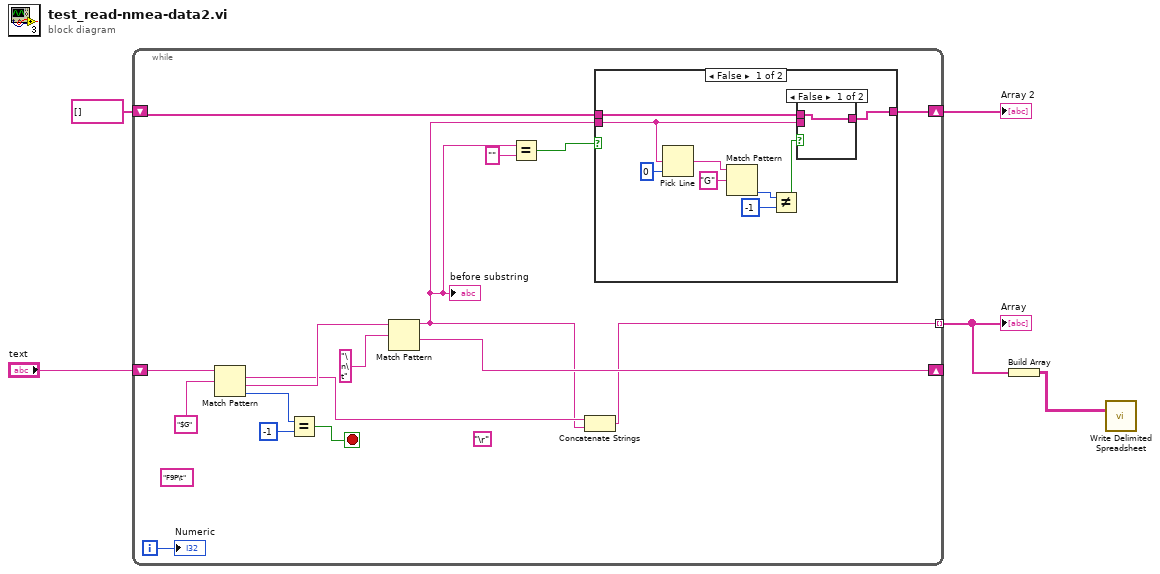
[diagram p0: block diagram]
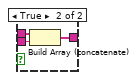
[diagram p2: hidden frame]
diagram:
  n1 = while {
    shift-right: [w15] -> _
    shift-left: "text" -> [w21]
    tunnel: [w6] -> w4 mode=indexing
    shift-right: [w11] -> w1
    shift-left: string[] [] -> [w12]
    i -> [w13]
    stop <- w14 stop-if-true
    (unwired) "\r"
    (unwired) "F9P\t" ("regular expression")
    n2 = Match Pattern(string=w21, regular expression="$G") -> (match substring=w8:string, after substring=w17:string, offset past match=w19:i32)  [unwired: 1 in, 1 out]
    n3 = Equal?(x=w19, y=-1) -> (x = y?=w14:bool)
    n4 = Match Pattern(string=w17, regular expression="\n\t") -> (before substring=w7:string, after substring=w15:string)  [unwired: 1 in, 2 out]
    "before substring" <- w7
    n5 = Equal?(x=w7, y="") -> (x = y?=w9:bool)
    n6 = Concatenate Strings(w8, w7) -> (w6:string)
    n7 = case shown="False" w9 {
      tunnel: w12 -> [w30 w35]
      tunnel: w7 -> [w28 _]
      tunnel: [w29 w35] -> w11
      frame False {
        n8 = Pick Line(multi-line string=w28, line index=0) -> (output string=w26:string)  [unwired: 1 in]
        n9 = Match Pattern(string=w26, regular expression="G") -> (offset past match=w24:i32)  [unwired: 1 in, 3 out]
        n10 = Not Equal?(x=w24, y=-1) -> (x != y?=w22:bool)
        n11 = case shown="False" w22 {
          tunnel: w30 -> [w31 w34]
          tunnel: [w31 w33] -> w29
          tunnel: w28 -> [_ w32]
          frame False {
          }
          frame True {
            n12 = Build Array (concatenate)(w34, w32) -> (w33:string[])
          }
        }
      }
      frame True {
      }
    }
    "Numeric" <- w13
  }
  "Array" <- w4
  "Array 2" <- w1
  n13 = Build Array(w4) -> (w3:string[][])
  n14 = call-poly <vilib>:"Write Delimited Spreadsheet.vi"("2D data"=w3) -> ()  [unwired: 13 in, 2 out]
